vi "HFRR ADV v020 new software.vi"() -> ()   [LabVIEW 2025] (continued)
            n2967 = call <vilib>:"Read Characters From File.vi"("file path (dialog if empty)"=w3832, "start of read offset (chars.:0)"=60 ("start of read offset (chars.: 0)")) -> ("character string"=→"String Control 4":string)  [unwired: 4 in, 3 out]
          }
        }
        n2968 = case shown="True" "OPEN 3" {
          frame False {
          }
          frame True {
            (unwired) 0  # existing file
            w3858 = "Choose a datalog file to open"  # prompt
            n2969 = local write "OPEN 3"(FALSE ("OPEN 1")) -> ()
            n2970 = String To Path(string="C:\\LAB-IQ\\Data\\") -> (path=w3843:path)
            n2971 = File Dialog(6:"*.dgf" ("pattern"), 7:w3858, 11:w3843) -> (0:w3841:errorcluster, 3:w3849:path)  [unwired: 4 in, 2 out]
            n2972 = Unbundle(w3841) -> ()  [unwired: 3 out]
            n2973 = Strip Path(path=w3849) -> (name=w3847:string)  [unwired: 1 out]
            n2974 = Path To String(path=w3849) -> (string=w3844:string)
            "string1 3" <- w3844
            n2975 = Match Pattern(string=w3847, regular expression=".dgf") -> (before substring=→"String Control 5":string)  [unwired: 1 in, 3 out]
            n2976 = Match Pattern(string=w3844, regular expression=".dgf" ("substring (\"\")")) -> (before substring=w3854:string)  [unwired: 1 in, 3 out]
            n2977 = Concatenate Strings(w3854, ".duf" ("Substring")) -> (w3851:string)
            n2978 = String To Path(string=w3851) -> (path=w3855:path)
            n2979 = call <vilib>:"Read Characters From File.vi"("file path (dialog if empty)"=w3855, "start of read offset (chars.:0)"=60 ("start of read offset (chars.: 0)")) -> ("character string"=→"String Control 6":string)  [unwired: 4 in, 3 out]
          }
        }
        n2980 = case shown="True" "OPEN 4" {
          frame False {
          }
          frame True {
            (unwired) 0  # existing file
            w3876 = "Choose a datalog file to open"  # prompt
            n2981 = local write "OPEN 4"(FALSE ("OPEN 1")) -> ()
            n2982 = String To Path(string="C:\\LAB-IQ\\Data\\") -> (path=w3861:path)
            n2983 = File Dialog(6:"*.dgf" ("pattern"), 7:w3876, 11:w3861) -> (0:w3859:errorcluster, 3:w3867:path)  [unwired: 4 in, 2 out]
            n2984 = Unbundle(w3859) -> ()  [unwired: 3 out]
            n2985 = Strip Path(path=w3867) -> (name=w3865:string)  [unwired: 1 out]
            n2986 = Path To String(path=w3867) -> (string=w3862:string)
            "string1 4" <- w3862
            n2987 = Match Pattern(string=w3865, regular expression=".dgf") -> (before substring=→"String Control 7":string)  [unwired: 1 in, 3 out]
            n2988 = Match Pattern(string=w3862, regular expression=".dgf" ("substring (\"\")")) -> (before substring=w3872:string)  [unwired: 1 in, 3 out]
            n2989 = Concatenate Strings(w3872, ".duf" ("Substring")) -> (w3869:string)
            n2990 = String To Path(string=w3869) -> (path=w3873:path)
            n2991 = call <vilib>:"Read Characters From File.vi"("file path (dialog if empty)"=w3873, "start of read offset (chars.:0)"=60 ("start of read offset (chars.: 0)")) -> ("character string"=→"String Control 8":string)  [unwired: 4 in, 3 out]
          }
        }
      }
      frame "About" {
        # "Elapsed time\ncof\nstroke\nmean pos\nTemp\nHumidity"
        n2992 = disable-structure shown="Disabled" {
          frame Disabled {
            n2993 = case shown="True" "Export" {
              frame False {
              }
              frame True {
                w3898 = "                                      " ("string")
                w3900 = "\r"
                (unwired) i16 6 ("width (-)")
                w3977 = "\r"
                w3909 = "\r"
                n2994 = local write "Export"(FALSE ("Export")) -> ()
                n2995 = local read "String 29"() -> (w3946:string)
                n2996 = local read "String 34"() -> (w3934:string)
                n2997 = local read "String 35"() -> (w3929:string)
                n2998 = local read "String 37"() -> (w3925:string)
                n2999 = local read "String 36"() -> (w3922:string)
                n3000 = local read "String 38"() -> (w3919:string)
                n3001 = local read "String 39"() -> (w3916:string)
                n3002 = Match Pattern(string=w3946, regular expression=".dwm") -> (before substring=w3942:string)  [unwired: 1 in, 3 out]
                "before substring" <- w3942
                n3003 = local read "S 38"() -> (w3937:string)
                n3004 = local read "S 39"() -> (w3930:string)
                n3005 = local read "Temperature before test 2"() -> (w3966:dbl)
                n3006 = local read "Temperature after test 2"() -> (w3971:dbl)
                n3007 = local read "Humidity before test 2"() -> (w3952:dbl)
                n3008 = local read "Humidity after test 2"() -> (w3967:dbl)
                n3009 = local read "MWSD 2"() -> (w3963:dbl)
                n3010 = local read "WS1.4 2"() -> (w3979:dbl)
                n3011 = local read "HCF 2"() -> (w3975:dbl)
                n3012 = local read "AVP 2"() -> (w3964:dbl)
                n3013 = Concatenate Strings("1," ("string"), w3937) -> (w3936:string)
                n3014 = Concatenate Strings("2," ("string"), w3934) -> (w3933:string)
                n3015 = Concatenate Strings("3," ("string"), w3930) -> (w3932:string)
                n3016 = Concatenate Strings("4," ("string"), w3929) -> (w3928:string)
                n3017 = Concatenate Strings("5," ("string"), w3925) -> (w3926:string)
                n3018 = Concatenate Strings("6," ("string"), w3922) -> (w3923:string)
                n3019 = Concatenate Strings("7," ("string"), w3919) -> (w3920:string)
                n3020 = Concatenate Strings("8," ("string"), w3916) -> (w3917:string)
                n3021 = local read "Sample ID"() -> (w3984:string)
                n3022 = case shown="\"xlx\"" "Select File Type" {
                  tunnel: w3942 -> [w3987 w3989 w3991]
                  tunnel: [w3985 w3990 w3992] -> w3941
                  frame "xlx" {
                    n3023 = Concatenate Strings(w3987, ".xls" ("string")) -> (w3985:string)
                  }
                  frame "csv" {
                    n3024 = Concatenate Strings(w3989, ".csv" ("string")) -> (w3990:string)
                  }
                  frame "txt" {
                    n3025 = Concatenate Strings(w3991, ".txt" ("string")) -> (w3992:string)
                  }
                }
                n3026 = local read "Test Date"() -> (w3983:string)
                n3027 = local read "String 45"() -> (w3897:string)
                n3028 = local read "String 31"() -> (w3982:string)
                n3029 = local read "String 32"() -> (w3981:string)
                n3030 = local read "TITTLE"() -> (w3905:string)
                n3031 = Number To Fractional String(number=w3952, width (-)=i16 6, precision (6)=i16 2) -> (F-format string=w3951:string)  [unwired: 1 in]
                n3032 = Number To Fractional String(number=w3966, width (-)=i16 6, precision (6)=i16 2) -> (F-format string=w3972:string)  [unwired: 1 in]
                n3033 = Number To Fractional String(number=w3967, width (-)=i16 6, precision (6)=i16 2) -> (F-format string=w3965:string)  [unwired: 1 in]
                n3034 = Number To Fractional String(number=w3971, width (-)=i16 6, precision (6)=i16 2) -> (F-format string=w3970:string)  [unwired: 1 in]
                n3035 = Number To Fractional String(number=w3963, width (-)=i16 6, precision (6)=i16 2) -> (F-format string=w3961:string)  [unwired: 1 in]
                n3036 = Number To Fractional String(number=w3964, width (-)=i16 6, precision (6)=i16 2) -> (F-format string=w3962:string)  [unwired: 1 in]
                n3037 = Number To Fractional String(number=w3975, width (-)=i16 6, precision (6)=i16 2) -> (F-format string=w3976:string)  [unwired: 1 in]
                n3038 = Number To Fractional String(number=w3979, precision (6)=i16 2) -> (F-format string=w3980:string)  [unwired: 2 in]
                n3039 = local read "s.NO"() -> (w3899:string)
                n3040 = Concatenate Strings("=" ("string"), w3905) -> (w3904:string)
                n3041 = Concatenate Strings("S.No," ("string"), "                                       Parameters" ("string")) -> (w3910:string)
                n3042 = Concatenate Strings(w3977, w3936, w3951, w3977, w3933, w3972, w3977, w3932, w3965, w3977, w3928, w3970, w3977, w3926, w3961, w3977, w3923, w3962, w3977, w3920, w3976, w3977, w3917, w3980) -> (w3939:string)
                n3043 = Concatenate Strings(w3909, "," ("string"), w3897, w3899, w3898, w3981, w3984, w3898, w3982, w3983, w3909) -> (w3907:string)
                n3044 = local read "Tested by"() -> (w3913:string)
                n3045 = local read "String 33"() -> (w3914:string)
                n3046 = Concatenate Strings("," ("string"), "                                                                             " ("string")) -> (w3902:string)
                n3047 = Concatenate Strings(w3904, w3900, w3907, w3900, w3910, w3939, w3900, w3902, w3914, w3913) -> (→"export":string)
                n3048 = String To Path(string=w3941) -> (path=w3948:path)
                n3049 = local read "export"() -> (w3943:string)
                n3050 = call <vilib>:"Write Characters To File.vi"("append to file? (new file:F)"=FALSE, "character string"=w3943, "file path (dialog if empty)"=w3948) -> ()  [unwired: 2 in, 1 out]
              }
            }
          }
          frame Enabled {
          }
        }
        n3051 = case shown="True" "OK Button 17" {
          frame False {
          }
          frame True {
            (unwired) 0  # existing file
            w4201 = "Choose a datalog file to open"  # prompt
            n3052 = local write "OK Button 17"(FALSE ("OK Button 17")) -> ()
            n3053 = local read "String"() -> (w4196:string)
            n3054 = String To Path(string=w4196) -> (path=w4197:path)
            n3055 = File Dialog(6:"*.duf" ("pattern"), 7:w4201, 11:w4197) -> (0:w4188:errorcluster, 3:w4207:path)  [unwired: 4 in, 2 out]
            n3056 = Unbundle(w4188) -> ()  [unwired: 3 out]
            n3057 = Open/Create/Replace File "Open File"(file path (use dialog)=w4207) -> (refnum out=w4199:refnum<file>)  [unwired: 5 in, 2 out]
            n3058 = Strip Path(path=w4207) -> (name=w4205:string)  [unwired: 1 out]
            n3059 = Path To String(path=w4207) -> (string=w4190:string)
            n3060 = while {
              tunnel: w4199 -> [w4211]
              i -> [w4208]
              stop <- w4209 continue-if-true
              (unwired) TRUE ("line mode (F)")
              n3061 = Read from Text File "Read File"(file (use dialog)=w4211) -> (text=w4210:string)  [unwired: 3 in, 3 out]
              n3062 = local write "Numeric 16"(w4208) -> ()
              n3063 = String Length(string=w4210) -> (length=w4213:i32)
              n3064 = Greater?(x=w4213, y=1) -> (0:w4209:bool)
            }
            n3065 = local write "String 29"(w4190) -> ()
            n3066 = Search and Replace String(input string=w4190, search string=".duf", replace string=".dgf" ("replace string (\"\")")) -> (result string=→"String Indicator 4":string)  [unwired: 5 in, 3 out]
            n3067 = Match Pattern(string=w4205, regular expression=".dwm") -> (before substring=w4189:string)  [unwired: 1 in, 3 out]
            "String Indicator" <- w4189
            n3068 = Match Pattern(string=w4190, regular expression=".dwm" ("substring (\"\")")) -> (before substring=w4191:string)  [unwired: 1 in, 3 out]
            "String Indicator 3" <- w4191
            n3069 = local write "TITTLE 2"(w4189) -> ()
            n3070 = String To Path(string=w4191) -> (path=w4198:path)
            "path" <- w4198
            n3071 = call <vilib>:"Read Characters From File.vi"("file path (dialog if empty)"=w4198, "start of read offset (chars.:0)"=60 ("start of read offset (chars.: 0)")) -> ("character string"=→"String Indicator 2":string)  [unwired: 4 in, 3 out]
          }
        }
        n3072 = call <vilib>:"Query Available Printers.vi"() -> ("system configured printers"=w3890:string[])  [unwired: 9 in, 2 out]
        "System Configured Printers 2" <- w3890
        n3073 = local read "OK Button 16"() -> (w3887:bool)
        n3074 = case shown="True" "OK Button 16" {
          frame False {
          }
          frame True {
            n3075 = stacked-sequence {
              frame #0 {
                n3076 = local read "Numeric 16"() -> (w4215:i32)
                n3077 = local write "Numeric 10"(w4215) -> ()
              }
              frame #1 {
                n3078 = local read "S.NO"() -> (→"s.NO":string)
                n3079 = local read "String 29"() -> (w4219:string)
                n3080 = String To Path(string=w4219) -> (path=w4218:path)
                n3081 = Open/Create/Replace File "Open File"(file path (use dialog)=w4218) -> (refnum out=w4220:refnum<file>)  [unwired: 5 in, 2 out]
                n3082 = for {
                  N: 16 -> [_]
                  tunnel: w4220 -> [w4227]
                  i -> [w4223]
                  (unwired) TRUE ("line mode (F)")
                  n3083 = Read from Text File "Read File"(file (use dialog)=w4227) -> (text=w4221:string)  [unwired: 3 in, 3 out]
                  n3084 = Match Pattern(string=w4221, regular expression="(") -> (after substring=w4226:string)  [unwired: 1 in, 3 out]
                  n3085 = Match Pattern(string=w4226, regular expression=")") -> (before substring=w4222:string)  [unwired: 1 in, 3 out]
                  n3086 = case shown="1" w4223 {
                    tunnel: w4222 -> [w4228 w4229 _ _ w4230 w4231 w4232 w4234 w4236 w4238 w4240 w4242 w4244 w4246 _]
                    tunnel: w4221 -> [_ _ _ _ _ _ _ _ _ _ _ _ _ _ _]
                    frame 0 {
                      "TITTLE" <- w4228
                    }
                    frame 1 {
                      "Sample ID" <- w4229
                    }
                    frame 2 {
                    }
                    frame 3 {
                    }
                    frame 4 {
                      "Test Date" <- w4230
                    }
                    frame 5 {
                      "Tested by" <- w4231
                    }
                    frame 6 {
                      n3087 = Fract/Exp String To Number(string=w4232) -> (number=→"Humidity before test 2":dbl)  [unwired: 3 in, 1 out]
                    }
                    frame 7 {
                      n3088 = Fract/Exp String To Number(string=w4234) -> (number=→"Temperature before test 2":dbl)  [unwired: 3 in, 1 out]
                    }
                    frame 8 {
                      n3089 = Fract/Exp String To Number(string=w4236) -> (number=→"Humidity after test 2":dbl)  [unwired: 3 in, 1 out]
                    }
                    frame 9 {
                      n3090 = Fract/Exp String To Number(string=w4238) -> (number=→"Temperature after test 2":dbl)  [unwired: 3 in, 1 out]
                    }
                    frame 10 {
                      n3091 = Fract/Exp String To Number(string=w4240) -> (number=→"MWSD 2":dbl)  [unwired: 3 in, 1 out]
                    }
                    frame 11 {
                      n3092 = Fract/Exp String To Number(string=w4242) -> (number=→"AVP 2":dbl)  [unwired: 3 in, 1 out]
                    }
                    frame 12 {
                      n3093 = Fract/Exp String To Number(string=w4244) -> (number=→"HCF 2":dbl)  [unwired: 3 in, 1 out]
                    }
                    frame 13 {
                      n3094 = Fract/Exp String To Number(string=w4246) -> (number=→"WS1.4 2":dbl)  [unwired: 3 in, 1 out]
                    }
                    frame 14, Default {
                    }
                  }
                }
              }
              frame #2 {
              }
            }
            n3095 = local write "OK Button 16"(FALSE ("OK Button 13")) -> ()
          }
        }
        n3096 = Index Array(array=w3890, index="Select Printer 3") -> (element=w3892:string)
        "Selected Printer" <- w3892
        n3097 = case shown="True" w3887 {
          frame False {
          }
          frame True {
            n3098 = flat-sequence {
              frame #0 {
              }
              frame #1 {
                n3099 = Wait (ms)(milliseconds to wait=u32 100) -> ()  [unwired: 1 out]
              }
              frame #2 {
                n3100 = local write "OK Button 16"(FALSE ("Print 3")) -> ()
              }
            }
          }
        }
        n3101 = case shown="True" "Print" {
          tunnel: w3892 -> [_ w4184]
          frame False {
          }
          frame True {
            (unwired) i16 6 ("width (-)")
            (unwired) "TESTED BY : "
            (unwired) "TESTED DATE :"
            (unwired) "SAMPLE ID : "
            (unwired) "SAMPLE DESIGN : "
            w4142 = "\r"
            w4159 = "\r"
            # "add image"
            n3102 = local read "Sample ID"() -> (w4132:string)
            n3103 = local read "Tested by"() -> (w4135:string)
            n3104 = local read "String 34"() -> (w4122:string)
            n3105 = local read "String 45"() -> (w4102:string)
            n3106 = local read "String 35"() -> (w4117:string)
            n3107 = local read "String 37"() -> (w4115:string)
            n3108 = local read "String 32"() -> (w4137:string)
            n3109 = local read "String 36"() -> (w4112:string)
            n3110 = local read "String 31"() -> (w4136:string)
            n3111 = local read "Test Date"() -> (w4133:string)
            n3112 = local read "String 33"() -> (w4138:string)
            n3113 = local read "String 38"() -> (w4108:string)
            n3114 = local read "String 39"() -> (w4105:string)
            n3115 = local write "Print"(FALSE ("Print FF")) -> ()
            n3116 = local read "S 39"() -> (w4120:string)
            n3117 = local read "S 38"() -> (w4127:string)
            n3118 = local read "Temperature before test 2"() -> (w4158:dbl)
            n3119 = local read "Temperature after test 2"() -> (w4148:dbl)
            n3120 = local read "Humidity before test 2"() -> (w4173:dbl)
            n3121 = local read "Humidity after test 2"() -> (w4157:dbl)
            n3122 = local read "MWSD 2"() -> (w4162:dbl)
            n3123 = local read "WS1.4 2"() -> (w4140:dbl)
            n3124 = Concatenate Strings("2)" ("string"), w4122) -> (w4123:string)
            n3125 = Concatenate Strings("3)" ("string"), w4120) -> (w4121:string)
            n3126 = Concatenate Strings("1)" ("string"), w4127) -> (w4126:string)
            n3127 = Concatenate Strings("4)" ("string"), w4117) -> (w4118:string)
            n3128 = Concatenate Strings("5)" ("string"), w4115) -> (w4114:string)
            n3129 = Concatenate Strings("6)" ("string"), w4112) -> (w4111:string)
            n3130 = Concatenate Strings("7)" ("string"), w4108) -> (w4109:string)
            n3131 = Concatenate Strings("8)" ("string"), w4105) -> (w4106:string)
            n3132 = local read "HCF 2"() -> (w4144:dbl)
            n3133 = local read "AVP 2"() -> (w4161:dbl)
            n3134 = local read "s.NO"() -> (w4103:string)
            n3135 = call <vilib>:"New Report.vi"("report type"=enum16{"Standard Report", "HTML"}."Standard Report") -> ("report out"=w4182:refnum<class "NI_report.lvclass">, "error out"=w4181:errorcluster)  [unwired: 13 in]
            n3136 = local read "TITTLE"() -> (w4134:string)
            n3137 = Concatenate Strings(w4159, w4102, w4103, w4159, w4137, w4132, w4159, w4136, w4133, w4159, w4138, w4135, w4159) -> (w4152:string)
            "test by" <- w4152
            n3138 = Number To Fractional String(number=w4158, width (-)=i16 6, precision (6)=i16 2) -> (F-format string=w4147:string)  [unwired: 1 in]
            n3139 = Number To Fractional String(number=w4157, width (-)=i16 6, precision (6)=i16 2) -> (F-format string=w4160:string)  [unwired: 1 in]
            n3140 = Number To Fractional String(number=w4173, width (-)=i16 6, precision (6)=i16 2) -> (F-format string=w4178:string)  [unwired: 1 in]
            n3141 = Number To Fractional String(number=w4162, width (-)=i16 6, precision (6)=i16 2) -> (F-format string=w4164:string)  [unwired: 1 in]
            n3142 = Number To Fractional String(number=w4148, width (-)=i16 6, precision (6)=i16 2) -> (F-format string=w4149:string)  [unwired: 1 in]
            n3143 = Number To Fractional String(number=w4161, width (-)=i16 6, precision (6)=i16 2) -> (F-format string=w4163:string)  [unwired: 1 in]
            n3144 = Number To Fractional String(number=w4144, width (-)=i16 6, precision (6)=i16 2) -> (F-format string=w4143:string)  [unwired: 1 in]
            n3145 = Number To Fractional String(number=w4140, precision (6)=i16 2) -> (F-format string=w4139:string)  [unwired: 2 in]
            n3146 = call-dynamic "Set Report Header Text.vi"("report in"=w4182, "center header text"=w4134, "error in (no error)"=w4181) -> ("report out"=w4153:refnum<class "NI_report.lvclass">, "error out"=w4154:errorcluster)  [unwired: 11 in]
            n3147 = Concatenate Strings(w4142, w4126, w4178, w4142, w4123, w4147, w4142, w4121, w4160, w4142, w4118, w4149, w4142, w4114, w4164, w4142, w4111, w4163, w4142, w4109, w4143, w4142, w4106, w4139) -> (w4130:string)
            "export 2" <- w4130
            n3148 = call-poly <vilib>:"Append Report Text.vi"("report in"=w4153, "text"=w4152, "error in (no error)"=w4154) -> ("report out"=w4156:refnum<class "NI_report.lvclass">, "error out"=w4155:errorcluster)  [unwired: 9 in, 2 out]
            n3149 = local read "test by"() -> (w4129:string)
            n3150 = local read "TITTLE"() -> (w4131:string)
            n3151 = call-poly <vilib>:"Append Report Text.vi"("report in"=w4156, "error in (no error)"=w4155) -> ("report out"=w4177:refnum<class "NI_report.lvclass">, "error out"=w4175:errorcluster)  [unwired: 10 in, 2 out]
            n3152 = Concatenate Strings(w4131, w4130, w4129) -> (→"output":string)
            n3153 = call-poly <vilib>:"Append Report Text.vi"("report in"=w4177, "text"=w4130, "error in (no error)"=w4175) -> ("report out"=w4176:refnum<class "NI_report.lvclass">, "error out"=w4174:errorcluster)  [unwired: 9 in, 2 out]
            n3154 = call-dynamic "Print Report.vi"("report in"=w4176, "printer name (default)"=w4184, "error in (no error)"=w4174) -> ("report out"=w4186:refnum<class "NI_report.lvclass">, "error out"=w4187:errorcluster)  [unwired: 11 in]
            n3155 = call-dynamic "Dispose Report.vi"("report in"=w4186, "error in (no error)"=w4187) -> ()  [unwired: 13 in, 1 out]
          }
        }
        n3156 = case shown="True" "Print 2" {
          frame False {
          }
          frame True {
            n3157 = flat-sequence {
              frame #0 {
                n3158 = local read "s.NO"() -> (→"s.NO 2":string)
                n3159 = Wait (ms)(milliseconds to wait=u32 20) -> ()  [unwired: 1 out]
                n3160 = local read "Sample ID  3"() -> (→"Sample ID  6":string)
                n3161 = local read "Sample ID  4"() -> (→"Sample ID  7":string)
                n3162 = local read "Sample ID"() -> (→"Sample ID  2":string)
                n3163 = local read "Tested by"() -> (→"Tested by 2":string)
                n3164 = local read "Test Date"() -> (→"Test Date 2":string)
                n3165 = local read "Humidity after test 3"() -> (→"Humidity after test 4":dbl)
                n3166 = local read "Ref A Test Date :"() -> (→"TITTLE 4":string)
                n3167 = local read "Temperature before test 3"() -> (w4009:dbl)
                n3168 = local read "Temperature before test 3"() -> (→"Temperature after test 5":dbl)
                n3169 = local read "Temperature after test 3"() -> (→"Temperature after test 4":dbl)
                n3170 = local read "Humidity before test 3"() -> (→"Humidity before test 4":dbl)
                n3171 = local write "Temperature before test 3"(w4009) -> ()
                n3172 = local read "image data"() -> (w4000:T16)
                n3173 = String To Path(string="C:\\LAB-IQ\\im\\Temp_resized.jpg") -> (path=w4001:path)
                "path 2" <- w4001
                n3174 = call <vilib>:"Write JPEG File.vi"("image data"=w4000, "path to JPEG file"=w4001) -> ()  [unwired: 8 in, 2 out]
                "Ref A Test Date :" <- "Ref A Test Date :"
                "Ref B Test Date :" <- "Ref B Test Date :"
                "Ref B Scar Value :" <- "Ref B Scar Value :"
                "Ref A Scar Value :" <- "Ref A Scar Value :"
              }
              frame #1 {
                (unwired) HTML_Report_Image_Alignment."MIDDLE" ("alignment (default)")
                w4037 = u16 0 items=["portrait", "landscape"] ("orientation (portrait)")
                (unwired) HTML_Report_Image_Alignment."ABSMIDDLE" ("alignment (default)")
                (unwired) "TESTED BY : "
                (unwired) "TESTED DATE :"
                (unwired) "SAMPLE ID : "
                (unwired) "SAMPLE DESIGN : "
                w4070 = "\r"
                # "add image"
                n3175 = Wait (ms)(milliseconds to wait=u32 20) -> ()  [unwired: 1 out]
                n3176 = local read "Sample ID  2"() -> (w4063:string)
                n3177 = local read "Wear Scar X"() -> (w4035:dbl)
                "Length ( microns ) 2" <- w4035
                n3178 = local read "Wear Scar Y"() -> (w4034:dbl)
                "Wear Scar Y ( microns ) :" <- w4034
                n3179 = local read "Test Date 2"() -> (w4064:string)
                n3180 = local read "Tested by 2"() -> (w4065:string)
                n3181 = local read "String 46"() -> (w4061:string)
                n3182 = local read "String 48"() -> (w4067:string)
                n3183 = local read "String 47"() -> (w4066:string)
                n3184 = local read "String 49"() -> (w4068:string)
                n3185 = local read "String 10"() -> (w4021:string)
                n3186 = local read "s.NO 2"() -> (w4062:string)
                n3187 = Add(x=w4035, y=w4034) -> (x+y=w4033:dbl)
                n3188 = call <vilib>:"New Report.vi"("report type"=enum16{"Standard Report", "HTML"}."HTML") -> ("report out"=w4041:refnum<class "NI_report.lvclass">, "error out"=w4039:errorcluster)  [unwired: 13 in]
                n3189 = Concatenate Strings(w4070, w4061, w4062, w4070, w4067, w4063, w4070, w4066, w4064, w4070, w4068, w4065, w4070) -> (→"test by 2":string)
                n3190 = Concatenate Strings("C:\\LAB-IQ\\Data\\" ("string"), w4021, ".jpg" ("string")) -> ()  [unwired: 1 out]
                n3191 = Divide(x=w4033, y=2.0) -> (x/y=→"Mean Wear ( microns) :":dbl)
                n3192 = call-dynamic "Set Report Orientation.vi"("report in"=w4041, "orientation (portrait)"=w4037, "error in (no error)"=w4039) -> ("report out"=w4040:refnum<class "NI_report.lvclass">, "error out"=w4038:errorcluster)  [unwired: 11 in]
                n3193 = for {
                  N: 5 -> [_]
                  tunnel: w4040 -> [w4091]
                  tunnel: [w4090] -> w4019
                  tunnel: w4038 -> [w4089]
                  tunnel: [w4088] -> w4018
                  n3194 = call-dynamic "Set Report Tab Width.vi"("report in"=w4091, "error in (no error)"=w4089) -> ("report out"=w4090:refnum<class "NI_report.lvclass">, "error out"=w4088:errorcluster)  [unwired: 12 in]
                }
                n3195 = local read "TITTLE"() -> (w4036:string)
                n3196 = call-dynamic "Set Report Header Text.vi"("report in"=w4019, "center header text"=w4036, "error in (no error)"=w4018) -> ("report out"=w4057:refnum<class "NI_report.lvclass">, "error out"=w4056:errorcluster)  [unwired: 11 in]
                n3197 = for {
                  N: 1 -> [_]
                  tunnel: [w4095] -> w4043
                  tunnel: [w4094] -> w4042
                  tunnel: w4057 -> [w4093]
                  tunnel: w4056 -> [w4092]
                  n3198 = call-dynamic "New Report Line.vi"("report in"=w4093, "error in (no error)"=w4092) -> ("report out"=w4095:refnum<class "NI_report.lvclass">, "error out"=w4094:errorcluster)  [unwired: 12 in]
                }
                n3199 = for {
                  N: 2 -> [_]
                  tunnel: [w4087] -> w4049
                  tunnel: [w4086] -> w4048
                  tunnel: w4043 -> [w4085]
                  tunnel: w4042 -> [w4084]
                  n3200 = call-dynamic "New Report Line.vi"("report in"=w4085, "error in (no error)"=w4084) -> ("report out"=w4087:refnum<class "NI_report.lvclass">, "error out"=w4086:errorcluster)  [unwired: 12 in]
                }
                n3201 = for {
                  N: 25 -> [_]
                  tunnel: w4049 -> [w4083]
                  tunnel: w4048 -> [w4081]
                  tunnel: [w4082] -> w4052
                  tunnel: [w4080] -> w4051
                  n3202 = call-dynamic "Set Report Tab Width.vi"("report in"=w4083, "error in (no error)"=w4081) -> ("report out"=w4082:refnum<class "NI_report.lvclass">, "error out"=w4080:errorcluster)  [unwired: 12 in]
                }
                n3203 = control-ref of="Tab Control 9"() -> (w4047:refnum<vi>)
                n3204 = call-dynamic "Append Control Image to Report.vi"("report in"=w4052, "alignment (default)"=HTML_Report_Image_Alignment."ABSMIDDLE", "ctrl reference"=w4047, "error in (no error)"=w4051) -> ("report out"=w4046:refnum<class "NI_report.lvclass">, "error out"=w4045:errorcluster)  [unwired: 8 in, 2 out]
                n3205 = for {
                  N: 3 -> [_]
                  tunnel: [w4079] -> w4030
                  tunnel: [w4078] -> w4029
                  tunnel: w4046 -> [w4077]
                  tunnel: w4045 -> [w4076]
                  n3206 = call-dynamic "New Report Line.vi"("report in"=w4077, "error in (no error)"=w4076) -> ("report out"=w4079:refnum<class "NI_report.lvclass">, "error out"=w4078:errorcluster)  [unwired: 12 in]
                }
                n3207 = for {
                  N: 100 -> [_]
                  tunnel: w4030 -> [w4075]
                  tunnel: w4029 -> [w4073]
                  tunnel: [w4074] -> w4026
                  tunnel: [w4072] -> w4024
                  n3208 = call-dynamic "Set Report Tab Width.vi"("report in"=w4075, "error in (no error)"=w4073) -> ("report out"=w4074:refnum<class "NI_report.lvclass">, "error out"=w4072:errorcluster)  [unwired: 12 in]
                }
                n3209 = String To Path(string="C:\\LAB-IQ\\im\\Temp_resized.jpg") -> (path=w4016:path)
                n3210 = call-poly <vilib>:"Append Image to Report.vi"("report in"=w4026, "path or URL of image"=w4016, "error in (no error)"=w4024) -> ("report out"=w4025:refnum<class "NI_report.lvclass">, "error out"=w4023:errorcluster)  [unwired: 9 in, 2 out]
                n3211 = call-poly <vilib>:"Open HTML Report in Browser.vi"("report in"=w4025, "error in (no error)"=w4023) -> ("report out"=w4060:refnum<class "NI_report.lvclass">, "error out"=w4059:errorcluster)  [unwired: 11 in, 1 out]
                n3212 = call-dynamic "Dispose Report.vi"("report in"=w4060, "error in (no error)"=w4059) -> ()  [unwired: 13 in, 1 out]
              }
              frame #2 {
              }
              frame #3 {
                n3213 = disable-structure shown="Disabled" {
                  frame Disabled {
                    n3214 = local read "String 10"() -> (w4100:string)
                    n3215 = Concatenate Strings("C:\\LAB-IQ-NXT\\Data\\" ("string"), w4100, ".jpg" ("string")) -> (w4098:string)
                    n3216 = String To Path(string=w4098) -> (path=w4097:path)
                    n3217 = Delete(path (use dialog)=w4097) -> ()  [unwired: 4 in, 3 out]
                  }
                  frame Enabled {
                  }
                }
                n3218 = local write "Print 2"(FALSE ("Print")) -> ()
              }
            }
          }
        }
      }
    }
    n3219 = property on="SetTemp" class="DigNum (strict)"("Disabled"=w2036) -> ()  [unwired: 2 in, 2 out]
    n3220 = Multiply(x=w2026, y=w2028) -> (x*y=w2027:dbl)
    n3221 = local read "MWSD"() -> (w2025:dbl)
    n3222 = Add(x=w2027, y=w2025) -> (x+y=→"WS1.4":dbl)
    n3223 = Wait (ms)(milliseconds to wait=u32 50) -> ()  [unwired: 1 out]
    n3224 = Wait (ms)(milliseconds to wait=u32 50) -> ()  [unwired: 1 out]
    n3225 = local read "Quit"() -> (w2024:bool)
  }
  n3226 = VISA Close(VISA resource name=w43, error in (no error)=w42) -> ()  [unwired: 1 out]
  n3227 = while {
    tunnel: [w4261] -> w52
    shift-right: [w4254] -> _
    shift-left: 0.0 -> [w4257]
    shift-right: [w4253] -> _
    shift-left: 0.0 -> [w4256]
    shift-right: [w4252] -> _
    shift-left: 400.0 ("vc_cmd") -> [w4255]
    stop <- w4261 stop-if-true
    # "PID LOGIC"
    n3228 = local read "RUN"() -> (w4259:bool)
    n3229 = local read "Auto Start Temp"() -> (w4248:bool)
    n3230 = local read "Auto Start Test"() -> (w4258:bool)
    n3231 = local read "START TEMP"() -> (w4250:bool)
    n3232 = And(x=w4248, y=w4258) -> (x .and. y?=w4249:bool)
    n3233 = Or(x=w4259, y=w4249) -> (x .or. y?=w4260:bool)
    n3234 = And(x=w4260, y=w4250) -> (x .and. y?=w4251:bool)
    n3235 = Wait (ms)(milliseconds to wait=u32 20) -> ()  [unwired: 1 out]
    n3236 = case shown="True" w4251 {
      tunnel: [400.0 ("out_vc_cmd") w4281] -> w4252
      tunnel: [w4264 w4283] -> w4253
      tunnel: [w4264 w4282] -> w4254
      tunnel: w4257 -> [_ w4272]
      tunnel: w4256 -> [_ w4271]
      tunnel: w4255 -> [_ w4270]
      frame False {
        w4264 = 0.0 ("error_out")
      }
      frame True {
        n3237 = local read "Set Strk"() -> (w4267:dbl)
        n3238 = local read "LVDT STROKE"() -> (w4265:dbl)
        n3239 = Add(x=w4267, y="Add up Stroke") -> (x+y=w4268:dbl)
        n3240 = formula code="// Zero-Hardcode Explicit Positional-Form PID Engine\n// Inputs: target_stroke, measured_stroke, dt, prev_error, integral_accumulator_in, prev_vc_cmd\n//         kp, ki, kd, max_step_change, max_amplitude, min_amplitude, startup_cmd\n// Outputs: vc_cmd, error_out, out_error, integral_accumulator_out, out_vc_cmd\n\n// 1. Calculate Tracking Error\nfloat current_error = target_stroke - measured_stroke;\nerror_out = current_error;\n\n// 2. Compute Proportional Term\nfloat p_term = kp * current_error;\n\n// 3. Compute Derivative Term\nfloat d_term = 0.0;\nif (dt > 0.0) {\n    d_term = kd * ((current_error - prev_error) / dt);\n}\n\n// 4. Update and Accumulate Integral Term\nfloat current_integral = integral_accumulator_in + (current_error * dt);\nfloat i_term = ki * current_integral;\n\n// 5. Calculate Ideal Target Command\nfloat ideal_command = startup_cmd + p_term + i_term + d_term;\n\n// 6. Anti-Windup Protection (Back-calculation method)\nif (ideal_command > max_amplitude) {\n    float excess = ideal_command - max_amplitude;\n    if (ki > 0.0) {\n        current_integral -= excess / ki;\n    }\n    ideal_command = max_amplitude;\n} else if (ideal_command < min_amplitude) {\n    float excess = ideal_command - min_amplitude;\n    if (ki > 0.0) {\n        current_integral -= excess / ki;\n    }\n    ideal_command = min_amplitude;\n}\n\n// 7. Apply Loop Rate Limiting (Protects voice coil from large voltage steps)\nfloat raw_adjustment = ideal_command - prev_vc_cmd;\n\nif (raw_adjustment > max_step_change) {\n    raw_adjustment = max_step_change;\n} else if (raw_adjustment < -max_step_change) {\n    raw_adjustment = -max_step_change;\n}\n\nfloat next_vc_cmd = prev_vc_cmd + raw_adjustment;\n\n// Final Output Safety Safeguard Clamping\nif (next_vc_cmd > max_amplitude) {\n    next_vc_cmd = max_amplitude;\n} else if (next_vc_cmd < min_amplitude) {\n    next_vc_cmd = min_amplitude;\n}\n\n// 8. Map to Shift Registers for memory persistence\nvc_cmd = next_vc_cmd;\nout_error = current_error;                     \nintegral_accumulator_out = current_integral;  \nout_vc_cmd = next_vc_cmd;"("target_stroke"=w4268, "measured_stroke"=w4265, "dt"="dt", "integral_accumulator_in"=w4271, "prev_error"=w4272, "prev_vc_cmd"=w4270, "kp"="kp", "ki"="ki", "kd"="kd", "max_step_change"="max_step_change", "max_amplitude"="max_amplitude", "min_amplitude"="min_amplitude", "startup_cmd"="startup_cmd") -> ("vc_cmd"=w4287:dbl, "out_error"=w4282:dbl, "integral_accumulator_out"=w4283:dbl, "out_vc_cmd"=w4281:dbl)  [unwired: 1 out]
        "output Vpp" <- w4287
        n3241 = Number To Fractional String(number=w4287, precision (6)=i16 1) -> (F-format string=w4285:string)  [unwired: 2 in]
        n3242 = Concatenate Strings("DAC;" ("string"), w4285) -> (w4269:string)
        n3243 = local write "Command"(w4269) -> ()
        "prev_error" <- w4272
        "integral_accumulator_in" <- w4271
        "prev_vc_cmd" <- w4270
      }
    }
    n3244 = local read "Quit"() -> (w4261:bool)
  }
  n3245 = Or(x=w48, y=w47) -> (x .or. y?=w49:bool)
  n3246 = Or(x=w45, y=w49) -> (x .or. y?=w54:bool)
  n3247 = control-ref of="new picture"() -> ()  [unwired: 1 out]
  n3248 = Or(x=w57, y=w54) -> (x .or. y?=w51:bool)
  n3249 = Or(x=w51, y=w52) -> (x .or. y?=w46:bool)
  n3250 = while {
    tunnel: [w4288] -> w56
    i -> [w4295]
    stop <- w4288 stop-if-true
    n3251 = local read "Quit"() -> (w4288:bool)
    n3252 = Equal To 0?(x=w4295) -> (x = 0?=w4293:bool)
    n3253 = call "Elapsed Time3"("Time Target (s)"=45.0, "Auto Reset"=TRUE) -> ("Time has Elapsed"=w4292:bool)  [unwired: 10 in, 7 out]
    n3254 = Wait (ms)(milliseconds to wait=u32 50) -> ()  [unwired: 1 out]
    n3255 = Or(x=w4292, y=w4293) -> (x .or. y?=w4294:bool)
    n3256 = case shown="True" w4294 {
      frame False {
      }
      frame True {
        n3257 = call <vilib>:"System Exec.vi"("run minimized? (F)"=TRUE, "error in (no error)"="error in (no error)", "command line"="powercfg.exe -change -monitor-timeout-ac 0") -> ("error out"=w4306:errorcluster)  [unwired: 5 in, 3 out]
        n3258 = call <vilib>:"System Exec.vi"("run minimized? (F)"=TRUE, "error in (no error)"=w4306, "command line"="powercfg.exe -change -disk-timeout-ac 0") -> ("error out"=w4305:errorcluster)  [unwired: 5 in, 3 out]
        n3259 = call <vilib>:"System Exec.vi"("run minimized? (F)"=TRUE, "error in (no error)"=w4305, "command line"="powercfg.exe -change -standby-timeout-ac 0") -> ("error out"=w4304:errorcluster)  [unwired: 5 in, 3 out]
        n3260 = call <vilib>:"System Exec.vi"("run minimized? (F)"=TRUE, "error in (no error)"=w4304, "command line"="powercfg.exe -change -hibernate-timeout-ac 0") -> ("error out"=w4303:errorcluster)  [unwired: 5 in, 3 out]
        n3261 = call <vilib>:"Simple Error Handler.vi"("error in (no error)"=w4303) -> ("error out"=w4309:errorcluster)  [unwired: 4 in, 4 out]
        n3262 = call <vilib>:"Clear Errors.vi"("error in (no error)"=w4309) -> ("error out"=→"error out":errorcluster)  [unwired: 5 in, 1 out]
      }
    }
  }
  n3263 = Compound Arithmetic op=OR(w59, w46, w56) -> (w58:bool)
  n3264 = flat-sequence {
    tunnel: w58 -> [_]
    tunnel: [w4311] -> w24
    tunnel: w24 -> [_]
    frame #0 {
      n3265 = call "CLOSE CONNECTION.vi"() -> ("error out"=w4311:errorcluster)  [unwired: 11 in]
    }
    frame #1 {
      n3266 = Quit LabVIEW(quit? (T)=TRUE) -> ()
      n3267 = local write "Quit"(FALSE ("EXIT")) -> ()
    }
  }
  n3268 = property on="Heater Button" class="Bool (strict)"("Visible"=TRUE) -> ()  [unwired: 2 in, 2 out]
  n3269 = disable-structure shown="Disabled" {
    disable-tunnel: _ -> [w4317 _]
    disable-tunnel: _ -> [w4314 _]
    disable-tunnel: _ -> [w4315 _]
    frame Disabled {
      n3270 = disable-structure shown="Disabled" {
        disable-tunnel: [w4324 _] -> w4316
        frame Disabled {
          n3271 = while {
            shift-right: [w4366] -> w4322
            shift-left: errorcluster {"status"=TRUE, "code"=0, "source"="Init"} ("error out") -> [w4331]
            shift-right: [w4365] -> w4321
            shift-left: _ -> [w4332]
            shift-right: [w4364] -> _
            shift-left: "" -> [w4363]
            tunnel: [w4325] -> w4324
            shift-right: ["Set Rh"] -> _
            shift-left: 0.0 ("Set Rh") -> [w4357]
            tunnel: [w4334] -> _
            i -> [w4334]
            stop <- w4325 stop-if-true
            n3272 = flat-sequence {
              tunnel: w4331 -> [w4369]
              tunnel: [w4369] -> w4330
              frame #0 {
                n3273 = Wait (ms)(milliseconds to wait=u32 200) -> ()  [unwired: 1 out]
              }
            }
            n3274 = local read "Com Port 3"() -> (w4333:refnum<visa-resource-name>)
            n3275 = local read "Humidity Str Rec"() -> (w4335:string)
            n3276 = Not Equal?(x="Set Rh", y=w4357) -> (x != y?=w4362:bool)
            n3277 = Number To Decimal String(number="Set Rh") -> (decimal integer string=w4360:string)  [unwired: 1 in]
            n3278 = Not Equal?(x=w4333, y=w4332) -> (x != y?=w4328:bool)
            n3279 = Concatenate Strings("#setPoint00" ("string"), w4360) -> (w4361:string)
            n3280 = case shown="False" w4362 {
              tunnel: w4361 -> [_ w4381]
              frame False {
                n3281 = local read "Humidity"() -> (w4378:bool)
                n3282 = case shown="True" w4378 {
                  frame False {
                    n3283 = local write "Humidity Str Send"("stop" ("Humidity Str Send")) -> ()
                  }
                  frame True {
                    n3284 = local write "Humidity Str Send"("start" ("Humidity Str Send")) -> ()
                  }
                }
              }
              frame True {
                n3285 = local write "Humidity Str Send"(w4381) -> ()
              }
            }
            n3286 = Or(x=w4328) -> (y=w4326:bool, x .or. y?=w4327:bool)
            n3287 = String Subset(string=w4335, offset (0)=7) -> (substring=w4350:string)  [unwired: 1 in]
            n3288 = Match Pattern(string=w4335, regular expression="?") -> (offset past match=w4353:i32)  [unwired: 1 in, 3 out]
            n3289 = Match Pattern(string=w4335, regular expression="v") -> (offset past match=w4356:i32)  [unwired: 1 in, 3 out]
            n3290 = case shown="True" w4327 {
              tunnel: w4330 -> [w4367 _]
              tunnel: [w4367 errorcluster {"status"=TRUE, "code"=0, "source"="Init"} ("error out")] -> w4329
              frame False {
              }
              frame True {
              }
            }
            n3291 = Equal?(x=w4353, y=-1) -> (x = y?=w4337:bool)
            n3292 = Match Pattern(string=w4350, regular expression="g") -> (after substring=w4351:string, offset past match=w4342:i32)  [unwired: 1 in, 2 out]
            n3293 = Match Pattern(string=w4350, regular expression="y") -> (after substring=w4349:string, offset past match=w4343:i32)  [unwired: 1 in, 2 out]
            n3294 = Greater?(x=w4343, y=w4342) -> (0:w4348:bool)
            n3295 = Greater Or Equal To 0?(x=w4343) -> (x >= 0?=w4340:bool)
            n3296 = Greater Or Equal To 0?(x=w4342) -> (x >= 0?=w4341:bool)
            n3297 = Or(x=w4340, y=w4341) -> (x .or. y?=w4339:bool)
            n3298 = Greater Or Equal To 0?(x=w4356) -> (x >= 0?=w4338:bool)
            n3299 = Select(t=w4349, s=w4348, f=w4351) -> (s? t:f=w4344:string)
            n3300 = case shown="Error" w4329 {
              selector: w4329 -> [w4394 w4440]
              tunnel: [w4392 w4433] -> w4366
              tunnel: w4332 -> [w4395 w4439]
              tunnel: [w4393 w4442] -> w4365
              tunnel: w4363 -> [w4382 w4441]
              tunnel: [w4389 w4441] -> w4364
              frame No Error {
                n3301 = call "Elapsed Time7"() -> ("Time has Elapsed"=w4388:bool)  [unwired: 12 in, 7 out]
                n3302 = Not Equal?(x="Humidity Str Send", y=w4382) -> (x != y?=w4384:bool)
                n3303 = Or(x=w4384, y=w4388) -> (x .or. y?=w4387:bool)
                n3304 = Select(t="Humidity Str Send", s=w4384, f="vals" ("regular expression")) -> (s? t:f=w4383:string)
                n3305 = Or(x=w4387, y="Send") -> (x .or. y?=w4391:bool)
                n3306 = case shown="True" w4391 {
                  tunnel: [w4398 w4403] -> w4392
                  tunnel: w4395 -> [w4397 w4411]
                  tunnel: w4394 -> [w4398 w4410]
                  tunnel: [w4397 w4404] -> w4393
                  tunnel: w4383 -> [_ w4409]
                  tunnel: [w4396 w4400] -> w4389
                  tunnel: "Humidity Str Send" -> [_ w4401]
                  tunnel: w4384 -> [_ w4402]
                  tunnel: w4382 -> [w4396 w4399]
                  frame False {
                  }
                  frame True {
                    n3307 = flat-sequence {
                      tunnel: w4411 -> [w4419]
                      tunnel: w4410 -> [w4418]
                      tunnel: w4409 -> [w4415]
                      tunnel: [w4417] -> w4408
                      tunnel: [w4416] -> w4407
                      tunnel: w4408 -> [w4422]
                      tunnel: w4407 -> [w4421]
                      tunnel: [w4422] -> w4406
                      tunnel: [w4421] -> w4405
                      tunnel: w4406 -> [w4429]
                      tunnel: w4405 -> [w4428]
                      tunnel: [w4427] -> w4404
                      tunnel: [w4426] -> w4403
                      frame #0 {
                        n3308 = local write "Ser Led"(TRUE ("Boolean 4")) -> ()
                        n3309 = Concatenate Strings(w4415, "\r") -> (w4414:string)
                        n3310 = VISA Write(VISA resource name=w4419, write buffer=w4414, error in (no error)=w4418) -> (VISA resource name out=w4417:refnum<visa-resource-name>, error out=w4416:errorcluster)  [unwired: 1 out]
                      }
                      frame #1 {
                        n3311 = Wait (ms)(milliseconds to wait="wait") -> ()  [unwired: 1 out]
                      }
                      frame #2 {
                        w4424 = FALSE ("Send")
                        n3312 = property class="Instr"(reference=w4429, error in=w4428) -> (reference out=w4430:refnum<visa-resource-name>, error out=w4431:errorcluster, "Serial Settings:Number of Bytes at Serial Port"=w4423:u32)
                        n3313 = local write "Send"(w4424) -> ()
                        n3314 = local write "Ser Led"(w4424) -> ()
                        n3315 = VISA Read(VISA resource name=w4430, byte count=w4423, error in (no error)=w4431) -> (VISA resource name out=w4427:refnum<visa-resource-name>, read buffer=→"Humidity Str Rec":string, error out=w4426:errorcluster)  [unwired: 1 out]
                      }
                    }
                    n3316 = Select(t=w4401, s=w4402, f=w4399) -> (s? t:f=w4400:string)
                  }
                }
              }
              frame Error {
                w4447 = u16 0 items=["None"=0, "XON/XOFF"=1, "RTS/CTS"=2, "DTR/DSR"=4] ("flow control")
                w4443 = u16 0 items=["None", "Odd", "Even", "Mark", "Space"] ("parity")
                w4446 = u16 10 items=["1.0"=10, "1.5"=15, "2.0"=20] ("stop bits")
                n3317 = VISA Close(VISA resource name=w4439, error in (no error)=w4440) -> (error out=w4438:errorcluster)
                n3318 = local write "humid"("" ("humid")) -> ()
                n3319 = local write "Humidity Str Rec"("" ("Humidity Str Rec")) -> ()
                n3320 = call <vilib>:"Clear Errors.vi"("error in (no error)"=w4438) -> ("error out"=w4437:errorcluster)  [unwired: 5 in, 1 out]
                n3321 = local read "Com Port 3"() -> (w4436:refnum<visa-resource-name>)
                n3322 = call-poly "VISA Configure Serial Port"("VISA resource name"=w4436, "timeout (10sec)"=u32 1000, "termination char\n(0xA = '\\n' = LF)"=u8 10 ("termination char\n(0xA = '\\n' = LF)"), "Enable Termination\nChar (T)"=FALSE ("Enable Termination Char (T)"), "data bits (8)"=u16 8 ("data bits"), "parity (0:none)"=w4443, "error in (no error)"=w4437, "stop bits (10: 1 bit)"=w4446, "flow control (0:none)"=w4447) -> ("VISA resource name out"=w4442:refnum<visa-resource-name>, "baud rate (9600)"=w4434:u32, "error out"=w4433:errorcluster)  [unwired: 4 in]
              }
            }
            n3323 = Compound Arithmetic op=AND(w4338, w4337, w4339) -> (w4336:bool)
            n3324 = case shown="True" w4336 {
              tunnel: w4335 -> [_ _]
              tunnel: w4344 -> [_ w4374]
              frame False {
              }
              frame True {
                w4372 = " " ("regular expression")
                n3325 = Match Pattern(string=w4374, regular expression=" ") -> (after substring=w4376:string)  [unwired: 1 in, 3 out]
                n3326 = Match Pattern(string=w4376, regular expression=w4372) -> (before substring=→"humid":string, after substring=w4373:string)  [unwired: 1 in, 2 out]
                n3327 = Match Pattern(string=w4373, regular expression=w4372) -> (before substring=→"temp_@Rh sensor":string)  [unwired: 1 in, 3 out]
              }
            }
            n3328 = local read "Quit"() -> (w4325:bool)
          }
          n3329 = VISA Close(VISA resource name=w4321, error in (no error)=w4322) -> (error out=w4318:errorcluster)
          n3330 = call <vilib>:"Clear Errors.vi"("error in (no error)"=w4318) -> ()  [unwired: 5 in, 2 out]
        }
        frame Enabled {
        }
      }
    }
    frame Enabled {
    }
  }
  n3331 = while {
    tunnel: [w4454] -> _
    i -> [w4454]
    stop <- w4450 stop-if-true
    # "Langauage selection"
    n3332 = Equal?(x="Lan flag", y=22.0) -> ()  [unwired: 1 out]
    n3333 = disable-structure shown="Disabled" {
      frame Disabled {
        n3334 = stacked-sequence {
          frame #0 {
            n3335 = case shown="\"Russian\"" "Language Selection" {
              tunnel: [0 1] -> w4456
              frame "English", Default {
              }
              frame "Russian" {
              }
            }
            n3336 = for {
              N: 130 -> [_]
              tunnel: "Table" -> [w4465]
              tunnel: w4456 -> [w4464]
              i -> [w4463]
              n3337 = Index Array(array=w4465, index (row)=w4463, index (col)=w4464) -> (element=w4462:string)
              n3338 = case shown="123" w4463 {
                tunnel: w4462 -> [w4466 w4467 _ w4468 w4469 w4470 w4471 w4472 w4473 w4474 w4475 w4476 w4477 w4478 w4479 w4480 w4481 w4482 w4483 w4484 w4485 w4486 w4487 w4488 w4489 w4490 w4491 w4492 w4493 _ _ w4494 w4495 w4496 w4497 w4498 w4499 w4508 w4515 w4522 w4529 w4533 w4536 w4539 w4541 w4543 w4544 w4545 w4546 w4547 w4548 w4549 w4550 w4551 w4552 w4553 w4554 w4555 w4556 w4557 w4558 w4559 w4560 w4561 w4562 w4563 w4564 w4565 w4566 w4567 w4568 w4569 w4570 w4571 w4572 w4573 w4574 w4575 w4576 w4577 w4578 w4579 w4580 w4581 w4582 w4583 w4584 w4585 w4586 w4587 w4588 w4589 w4590 w4591 w4592 w4593 w4594 w4595 w4596 w4597 w4598 w4599 w4600 w4601 w4602 _ w4603 w4604 w4605 w4606 w4607 w4608 w4609 w4610 w4611 w4612 w4613 w4614 w4615 _ w4616 w4617 w4618 w4619 w4620 w4621 _]
                frame 0 {
                  n3339 = local write "S"(w4466) -> ()
                }
                frame 1 {
                  n3340 = local write "S 2"(w4467) -> ()
                }
                frame 2 {
                }
                frame 3 {
                  n3341 = local write "S 4"(w4468) -> ()
                }
                frame 4 {
                  n3342 = property on="FILE" class="Str"("Caption.Text"=w4469) -> ()  [unwired: 2 in, 2 out]
                }
                frame 5 {
                  n3343 = property on="Fuel Discription :" class="Str"("Caption.Text"=w4470) -> ()  [unwired: 2 in, 2 out]
                }
                frame 6 {
                  n3344 = property on="Remarks :" class="Str"("Caption.Text"=w4471) -> ()  [unwired: 2 in, 2 out]
                }
                frame 7 {
                  n3345 = property on="Save & Continue" class="Bool (strict)"("Boolean Text.Text"=w4472) -> ()  [unwired: 2 in, 2 out]
                }
                frame 8 {
                }
                frame 9 {
                  n3346 = property on="Set Hz" class="DigNum (strict)"("Caption.Text"=w4474) -> ()  [unwired: 2 in, 2 out]
                }
                frame 10 {
                  "String 3" <- w4475
                }
                frame 11 {
                  n3347 = property on="NORMAL LOAD" class="DigNum (strict)"("Caption.Text"=w4476) -> ()  [unwired: 2 in, 2 out]
                }
                frame 12 {
                  "String 5" <- w4477
                }
                frame 13 {
                  n3348 = property on="Set Temp" class="DigNum (strict)"("Caption.Text"=w4478) -> ()  [unwired: 2 in, 2 out]
                }
                frame 14 {
                  n3349 = local write "S 15"(w4479) -> ()
                }
                frame 15 {
                  n3350 = property on="Set Rh" class="DigNum (strict)"("Caption.Text"=w4480) -> ()  [unwired: 2 in, 2 out]
                }
                frame 16 {
                  "String 13" <- w4481
                  "String 26" <- w4481
                }
                frame 17 {
                  n3351 = local write "S 18"(w4482) -> ()
                }
                frame 18 {
                  "String 17" <- w4483
                }
                frame 19 {
                  n3352 = property on="test time" class="DigNum (strict)"("Caption.Text"=w4484) -> ()  [unwired: 2 in, 2 out]
                }
                frame 20 {
                  "String 18" <- w4485
                  "String 22" <- w4485
                }
                frame 21 {
                  n3353 = property on="Elapsed time" class="DigNum (strict)"("Caption.Text"=w4486) -> ()  [unwired: 2 in, 2 out]
                }
                frame 22 {
                  n3354 = property on="Samplingtime 2" class="DigNum (strict)"("Caption.Text"=w4487) -> ()  [unwired: 2 in, 2 out]
                }
                frame 23 {
                  "String 21" <- w4488
                }
                frame 24 {
                  n3355 = property on="Countdown" class="DigNum (strict)"("Caption.Text"=w4489) -> ()  [unwired: 2 in, 2 out]
                }
                frame 25 {
                  n3356 = property on="Countdown 2" class="DigNum (strict)"("Caption.Text"=w4490) -> ()  [unwired: 2 in, 2 out]
                }
                frame 26 {
                  n3357 = property on="Engage" class="Bool (strict)"("Boolean Text.Text"=w4491) -> ()  [unwired: 2 in, 2 out]
                }
                frame 27 {
                  n3358 = property on="Boolean  4" class="Bool (strict)"("Boolean Text.Text"=w4492) -> ()  [unwired: 2 in, 2 out]
                }
                frame 28 {
                  n3359 = property on="Test \nStatus" class="Bool (strict)"("Boolean Text.Text"=w4493) -> ()  [unwired: 2 in, 2 out]
                }
                frame 29 {
                }
                frame 30 {
                }
                frame 31 {
                }
                frame 32 {
                  n3360 = property on="RSTCOF" class="Bool"("Boolean Text.Text"=w4495) -> ()  [unwired: 2 in, 2 out]
                  n3361 = property on="RST FF" class="Bool"("Boolean Text.Text"=w4495) -> ()  [unwired: 2 in, 2 out]
                  n3362 = property on="RST TEMP" class="Bool"("Boolean Text.Text"=w4495) -> ()  [unwired: 2 in, 2 out]
                  n3363 = property on="RSTV1 3" class="Bool"("Boolean Text.Text"=w4495) -> ()  [unwired: 2 in, 2 out]
                  n3364 = property on="rstv2" class="Bool"("Boolean Text.Text"=w4495) -> ()  [unwired: 2 in, 2 out]
                  n3365 = property on="RSTV1 2" class="Bool"("Boolean Text.Text"=w4495) -> ()  [unwired: 2 in, 2 out]
                  n3366 = property on="RST CP" class="Bool"("Boolean Text.Text"=w4495) -> ()  [unwired: 2 in, 2 out]
                }
                frame 33 {
                  "S 61" <- w4496
                }
                frame 34 {
                  "String 23" <- w4497
                }
                frame 35 {
                  n3367 = property on="Rh Before" class="DigNum (strict)"("Caption.Text"=w4498) -> ()  [unwired: 2 in, 2 out]
                }
                frame 36 {
                  n3368 = Match Pattern(string=w4499, regular expression=",") -> (before substring=→"bs":string, after substring=→"as":string)  [unwired: 1 in, 2 out]
                  n3369 = property on="Rh After" class="DigNum (strict)"("Caption.Text"=w4499) -> ()  [unwired: 2 in, 2 out]
                }
                frame 37 {
                  n3370 = Match Pattern(string=w4508, regular expression=",") -> (before substring=w4507:string, after substring=w4506:string)  [unwired: 1 in, 2 out]
                  "bs" <- w4507
                  "as" <- w4506
                  n3371 = Concatenate Strings(w4507, w4506) -> (w4503:string)
                  n3372 = property on="Humidity before test 2" class="DigNum (strict)"("Caption.Text"=w4503) -> ()  [unwired: 2 in, 2 out]
                  n3373 = property on="Humidity before test" class="DigNum (strict)"("Caption.Text"=w4503) -> ()  [unwired: 2 in, 2 out]
                  n3374 = Concatenate Strings(w4503, "=" ("string")) -> (w4504:string)
                  n3375 = local write "S 38"(w4504) -> ()
                }
                frame 38 {
                  n3376 = Match Pattern(string=w4515, regular expression=",") -> (before substring=w4514:string, after substring=w4513:string)  [unwired: 1 in, 2 out]
                  "bs" <- w4514
                  "as" <- w4513
                  n3377 = Concatenate Strings(w4514, w4513) -> (w4510:string)
                  n3378 = property on="Humidity after test 2" class="DigNum (strict)"("Caption.Text"=w4510) -> ()  [unwired: 2 in, 2 out]
                  n3379 = Concatenate Strings(w4510, "=" ("string")) -> (w4512:string)
                  n3380 = property on="Humidity after test" class="DigNum (strict)"("Caption.Text"=w4510) -> ()  [unwired: 2 in, 2 out]
                  n3381 = local write "S 39"(w4512) -> ()
                }
                frame 39 {
                  n3382 = Match Pattern(string=w4522, regular expression=",") -> (before substring=w4521:string, after substring=w4520:string)  [unwired: 1 in, 2 out]
                  "bs" <- w4521
                  "as" <- w4520
                  n3383 = Concatenate Strings(w4521, w4520) -> (w4517:string)
                  n3384 = property on="Temperature before test 2" class="DigNum (strict)"("Caption.Text"=w4517) -> ()  [unwired: 2 in, 2 out]
                  n3385 = property on="Temperature before test" class="DigNum (strict)"("Caption.Text"=w4517) -> ()  [unwired: 2 in, 2 out]
                  n3386 = Concatenate Strings(w4517, "=" ("string")) -> (→"String 34":string)
                }
                frame 40 {
                  n3387 = Match Pattern(string=w4529, regular expression=",") -> (before substring=w4528:string, after substring=w4527:string)  [unwired: 1 in, 2 out]
                  "bs" <- w4528
                  "as" <- w4527
                  n3388 = Concatenate Strings(w4528, w4527) -> (w4524:string)
                  n3389 = property on="Temperature after test 2" class="DigNum (strict)"("Caption.Text"=w4524) -> ()  [unwired: 2 in, 2 out]
                  n3390 = Concatenate Strings(w4524, "=" ("string")) -> (→"String 35":string)
                  n3391 = property on="Temperature after test" class="DigNum (strict)"("Caption.Text"=w4524) -> ()  [unwired: 2 in, 2 out]
                }
                frame 41 {
                  n3392 = property on="AVP" class="DigNum (strict)"("Caption.Text"=w4533) -> ()  [unwired: 2 in, 2 out]
                  n3393 = property on="AVP 2" class="DigNum (strict)"("Caption.Text"=w4533) -> ()  [unwired: 2 in, 2 out]
                  n3394 = Concatenate Strings(w4533, "=" ("string")) -> (→"String 36":string)
                }
                frame 42 {
                  n3395 = property on="MWSD" class="DigNum (strict)"("Caption.Text"=w4536) -> ()  [unwired: 2 in, 2 out]
                  n3396 = property on="MWSD 2" class="DigNum (strict)"("Caption.Text"=w4536) -> ()  [unwired: 2 in, 2 out]
                  n3397 = Concatenate Strings(w4536, "=" ("string")) -> (→"String 37":string)
                }
                frame 43 {
                  n3398 = property on="HCF 2" class="DigNum (strict)"("Caption.Text"=w4539) -> ()  [unwired: 2 in, 2 out]
                  n3399 = property on="HCF" class="DigNum (strict)"("Caption.Text"=w4539) -> ()  [unwired: 2 in, 2 out]
                  n3400 = Concatenate Strings(w4539, "=" ("string")) -> (→"String 38":string)
                }
                frame 44 {
                  n3401 = Concatenate Strings(w4541, "=" ("string")) -> (→"String 39":string)
                  n3402 = property on="WS1.4 2" class="DigNum (strict)"("Caption.Text"=w4541) -> ()  [unwired: 2 in, 2 out]
                  n3403 = property on="WS1.4" class="DigNum (strict)"("Caption.Text"=w4541) -> ()  [unwired: 2 in, 2 out]
                }
                frame 45 {
                  n3404 = property on="Save Results" class="Bool (strict)"("Boolean Text.Text"=w4543) -> ()  [unwired: 2 in, 2 out]
                }
                frame 46 {
                  n3405 = local write "S 47"(w4544) -> ()
                }
                frame 47 {
                  n3406 = local write "S 48"(w4545) -> ()
                }
                frame 48 {
                  n3407 = local write "S 49"(w4546) -> ()
                }
                frame 49 {
                  n3408 = local write "S 50"(w4547) -> ()
                }
                frame 50 {
                  n3409 = local write "S 51"(w4548) -> ()
                }
                frame 51 {
                  n3410 = local write "S 52"(w4549) -> ()
                }
                frame 52 {
                  n3411 = local write "S 53"(w4550) -> ()
                }
                frame 53 {
                  n3412 = local write "S 54"(w4551) -> ()
                }
                frame 54 {
                  n3413 = local write "S 55"(w4552) -> ()
                }
                frame 55 {
                  n3414 = local write "S 56"(w4553) -> ()
                }
                frame 56 {
                  n3415 = local write "S 57"(w4554) -> ()
                }
                frame 57 {
                  n3416 = local write "S 58"(w4555) -> ()
                }
                frame 58 {
